vi "Drive Get and use.vi"(0 "Slow Drive":bool, 1 "Y - Axis":dbl, 2 "X - Axis":dbl) -> ()   [LabVIEW 2013]
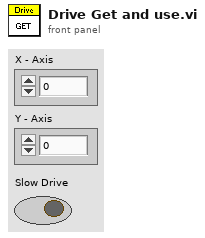
[diagram p1: front panel]
types:
  T1 = cluster{"Axis X":dbl, "Axis Y":dbl, "Slow Drive":bool}
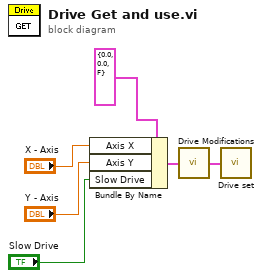
[diagram p0: block diagram]
diagram:
  n1 = Bundle By Name(cluster=T1 {"Axis X"=0.0, "Axis Y"=0.0, "Slow Drive"=FALSE} ("Drive Info"), "Axis X"="X - Axis", "Axis Y"="Y - Axis", "Slow Drive"="Slow Drive") -> (w2:T1)
  n2 = call "Drive Modifications.vi"("Drive Info In"=w2) -> ("Drive Info Out"=w3:T1)
  n3 = call "Drive set.vi"("Drive Info In"=w3) -> ()  [unwired: 1 out]
